vi "channel operation tests.vi"() -> (3 "channels match":bool)   [LabVIEW 2015, in "tdms logger tests.lvlib"]
uses:
  tdms logger tests.lvlib
  configuration/TDMS datalogger configuration.lvclass
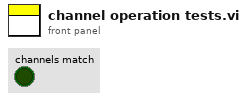
[diagram p1: front panel]
types:
  T1 = cluster{"channel":refnum<class "TBM channel.lvclass">}[]
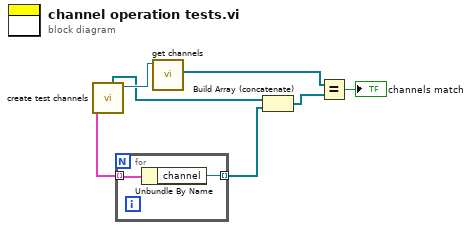
[diagram p0: block diagram]
diagram:
  n1 = call "create test channels.vi"() -> ("TDMS datalogger configuration out"=w5:refnum<class "TDMS datalogger configuration.lvclass">, "chans"=w3:refnum<class "TBM channel.lvclass">[], "Lines"=w4:T1)  [unwired: 3 in, 6 out]
  n2 = for {
    tunnel: w4 -> [w9] mode=indexing
    tunnel: [w8] -> w2 mode=indexing
    n3 = Unbundle By Name(w9) -> ("channel"=w8:refnum<class "TBM channel.lvclass">)
  }
  n4 = call-dynamic "get channels.vi"("module configuration in"=w5) -> ("channels"=w7:refnum<class "TBM channel.lvclass">[])  [unwired: 9 in, 1 out]
  n5 = Build Array (concatenate)(w3, w2) -> (w1:refnum<class "TBM channel.lvclass">[])
  n6 = Equal?(x=w7, y=w1) -> (x = y?=→"channels match":bool)
